vi "Get Disp Xml Data.vi"(8 "error in":errorcluster caption="Error In (no error)") -> (0 "error out":errorcluster caption="Error Out", 3 "DispXml[]":string[](array[string]))   [LabVIEW 2016]
uses:
  <vilib>/Pansino Software/LabVIEW Architecture/Queue Management/PSARC_Queue Create_Single.vi
  <vilib>/Pansino Software/LabVIEW Architecture/Queue Management/PSARC_Queue Insert Element.vi
  <vilib>/Pansino Software/LabVIEW Architecture/Queue Management/PSARC_Queue Remove Element.vi
  <vilib>/Pansino Software/LabVIEW Architecture/Queue Management/PSARC_Queue Destroy_Single.vi
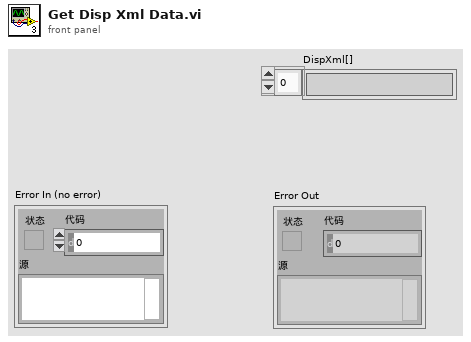
[diagram p1: front panel]
types:
  T1 = cluster{"Main Queue":string, "DAQ Queue":string, "ANA Queue":string, "CUI Queue":string, "Q-FocusList":string, "Q-Toolbar":string, "Q-Config":string}
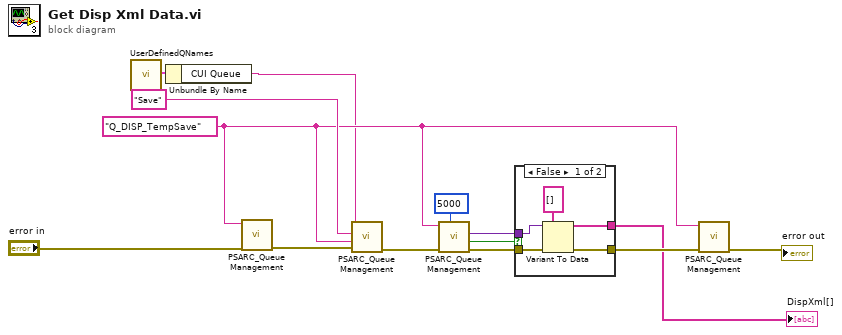
[diagram p0: block diagram]
diagram:
  w10 = "Q_DISP_TempSave" ("Queue Name")
  n1 = call "UserDefinedQNames.vi"() -> ("All Queues"=w2:T1)  [unwired: 11 in]
  n2 = Unbundle By Name(w2) -> ("CUI Queue"=w1:string)
  n3 = call-poly <vilib>:"PSARC_Queue Management.vi"("error in (no error)"="error in", "Queue Name"=w10) -> ("error out"=w14:errorcluster)  [unwired: 8 in, 1 out]
  n4 = call-poly <vilib>:"PSARC_Queue Management.vi"("error in (no error)"=w14, "Data"=w10, "Event"="Save", "Queue Name(unamed)"=w1) -> ("error out"=w12:errorcluster)  [unwired: 6 in, 1 out]
  n5 = call-poly <vilib>:"PSARC_Queue Management.vi"("Time out(-1)_queue out"=5000, "error in (no error)"=w12, "Queue Name(unamed)"=w10) -> ("error out"=w8:errorcluster, "timed out"=w6:bool, "Data"=w5:variant)  [unwired: 5 in, 1 out]
  n6 = case shown="False" w6 {
    tunnel: w8 -> [w19 w20]
    tunnel: [w18 w20] -> w7
    tunnel: w5 -> [w17 _]
    tunnel: [w15 _] -> w4
    frame False {
      n7 = Variant To Data(error in=w19, type=string[] [], Variant=w17) -> (data=w15:string[], error out=w18:errorcluster)
    }
    frame True {
    }
  }
  "DispXml[]" <- w4
  n8 = call-poly <vilib>:"PSARC_Queue Management.vi"("error in (no error)"=w7, "Queue Name(unamed)"=w10) -> ("error out"=→"error out":errorcluster)  [unwired: 7 in, 2 out]
